vi "Create calibration array.vi"() -> ()   [LabVIEW 2009, in "Varian Magnet.lvclass"]
uses:
  Varian Magnet.lvclass
panel:
  out "Calibration array":dbl[][](array[numeric])
  in  "Create calibration array":bool
  in  "stop":bool
  in  "step size":dbl[unit]
  in  "ending field":dbl[unit]
  in  "starting field":dbl[unit]
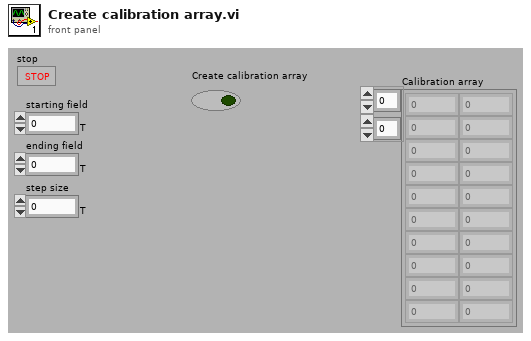
[diagram p1: front panel]
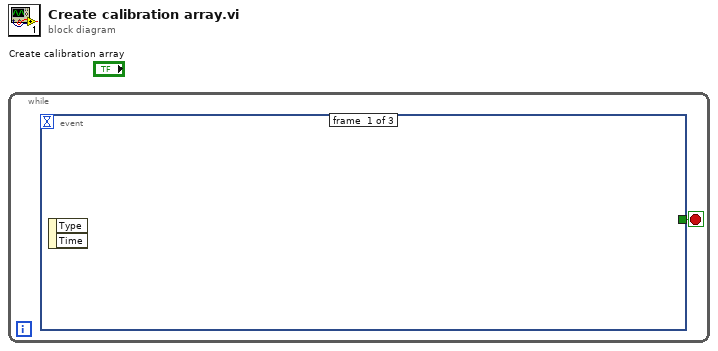
[diagram p0: block diagram]
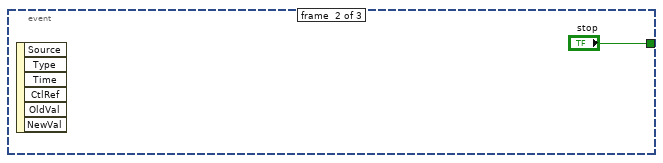
[diagram p2: hidden frame]
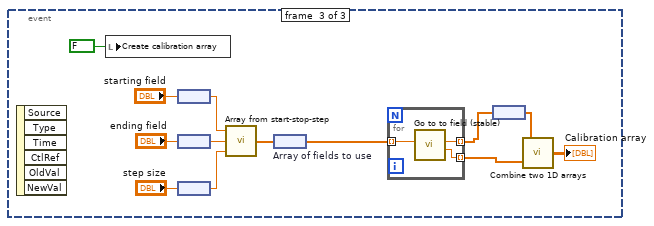
[diagram p3: hidden frame]
diagram:
  n1 = while {
    stop <- w1 stop-if-true
    n2 = event shown="[2] \"Create calibration array\": Value Change" {
      selector: _ -> [_ _ _]
      dyn-events: _ -> [_ _ _]
      timeout: _ -> [_ _ _]
      tunnel: [_ "stop" _] -> w1
      event #0 {
        n3 = event-data() -> ()  [unwired: 3 out]
      }
      event #1 {
        n4 = event-data() -> ()  [unwired: 7 out]
      }
      event #2 {
        n5 = event-data() -> ()  [unwired: 7 out]
        n6 = local write "Create calibration array"(FALSE ("Create calibration array")) -> ()
        n7 = node("starting field") -> (w9:dbl)
        n8 = node("ending field") -> (w12:dbl)
        n9 = node("step size") -> (w8:dbl)
        n10 = call "Array from start-stop-step.vi"("Step"=w8, "Stop"=w12, "Start"=w9) -> ("Array of numbers"=w10:dbl[])
        n11 = node "Array of fields to use"(w10) -> (w7:dbl[unit][])
        n12 = for {
          tunnel: w7 -> [w18] mode=indexing
          tunnel: [w17] -> w4 mode=indexing
          tunnel: [w16] -> w6 mode=indexing
          n13 = call "Go to to field (stable).vi"("Desired field"=w18) -> ("Current control voltage"=w16:dbl, "Current field"=w17:dbl[unit])  [unwired: 2 in, 7 out]
        }
        n14 = node(w4) -> (w3:dbl[])
        n15 = call "Combine two 1D arrays.vi"("Array2"=w6, "Array1"=w3) -> ("Combined array"=→"Calibration array":dbl[][])
      }
    }
  }
